vi "Dialog_SelectTarget.vi"(5 "error in (no error)":errorcluster) -> (15 "target address out":string, 16 "cancel?":bool, 17 "TCP port out":u16, 19 "error out":errorcluster)   [LabVIEW 2017, in "G#RemoteProxy.lvclass"]
doc: "Dialog that let you select the target to debug."
uses:
  G#RemoteProxy.lvclass
panel:
  in  "TCP Port":u16=62001
  in  "Available Targets":i32(ring) items=["My Computer (0.0.0.0)"]
  in  "TargetType":enum32{"Targets in project", "Specify"}(radio)
  in  "Cancel":bool
  in  "Specify target address":string
  in  "Connect":bool
  # "Select Target"
  # "Make sure that the\nG#DebugServer is running\non the remote target."
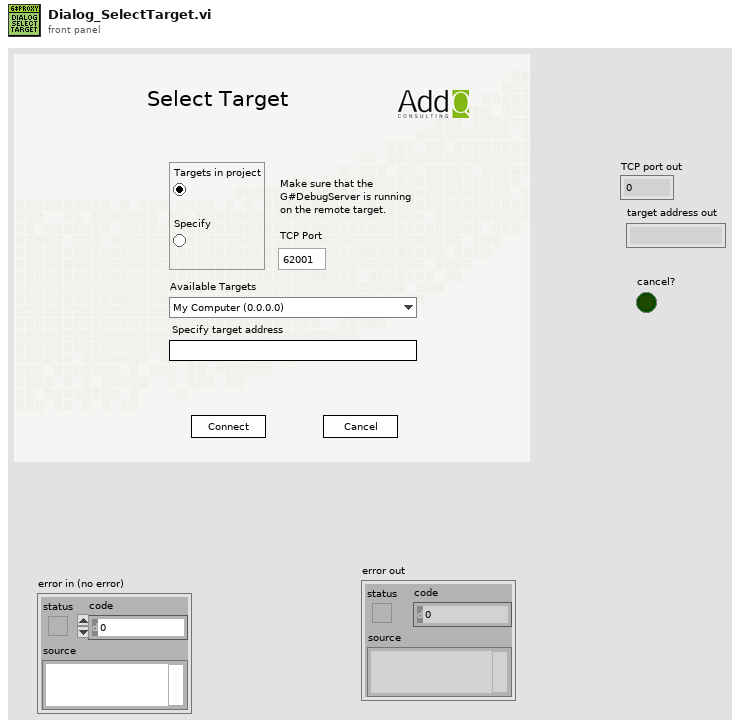
[diagram p1: front panel]
types:
  T1 = enum8{"Enabled", "Disabled", "Disabled and Grayed Out"}
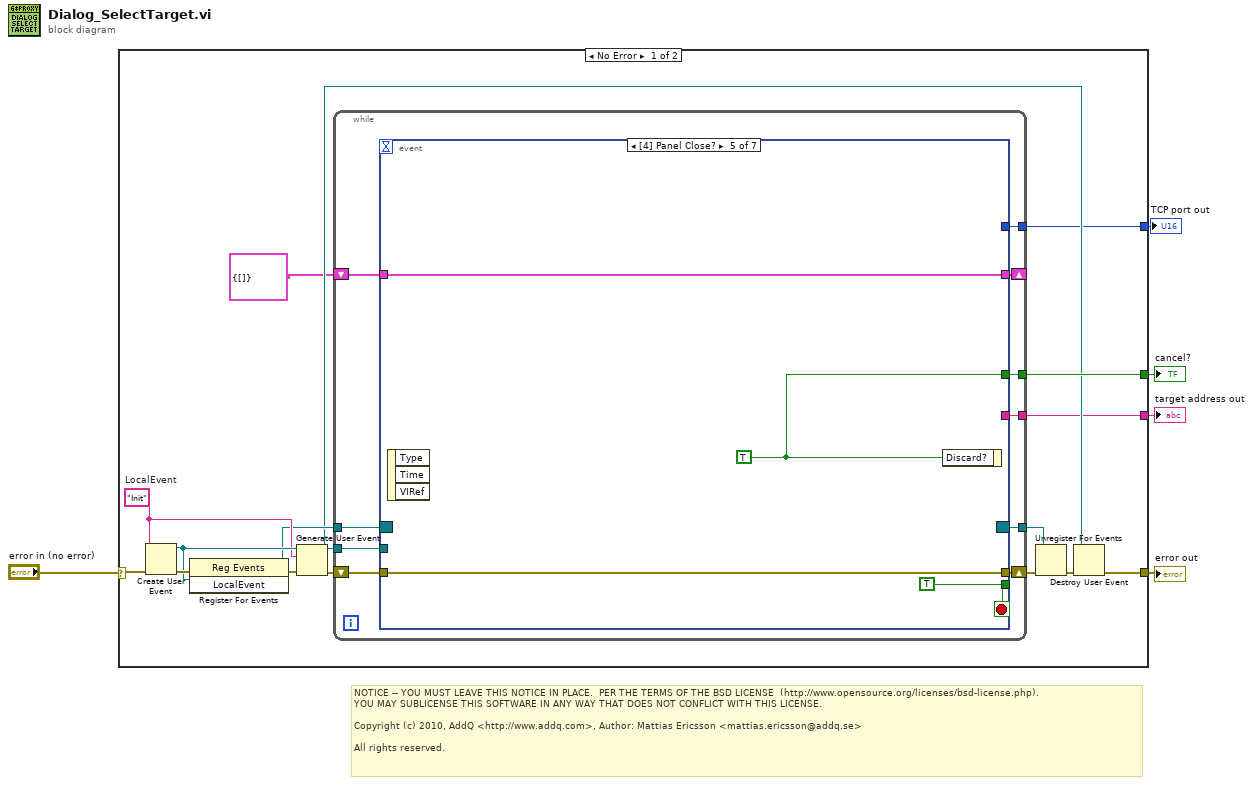
[diagram p0: block diagram]
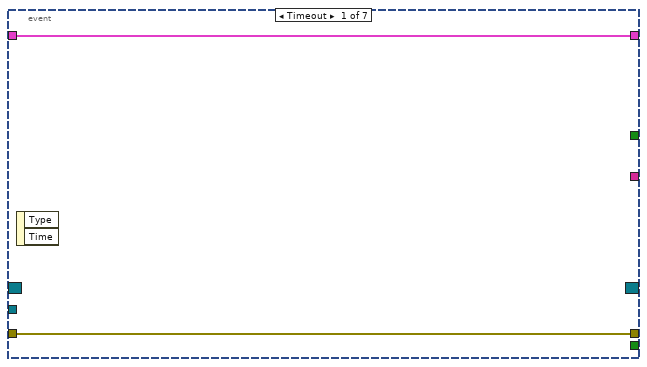
[diagram p2: hidden frame]
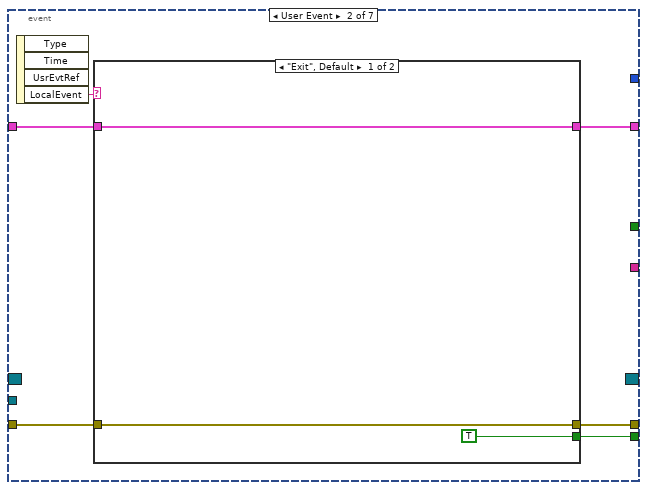
[diagram p3: hidden frame]
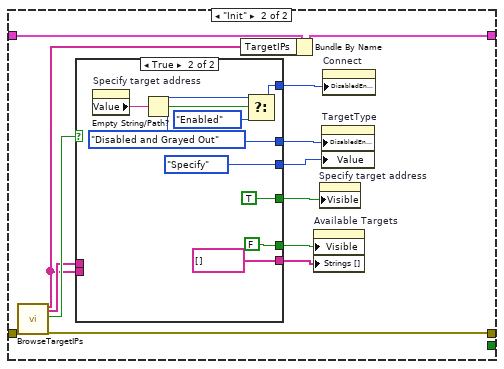
[diagram p4: hidden frame]
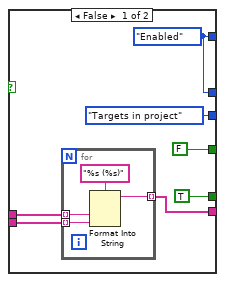
[diagram p5: hidden frame]
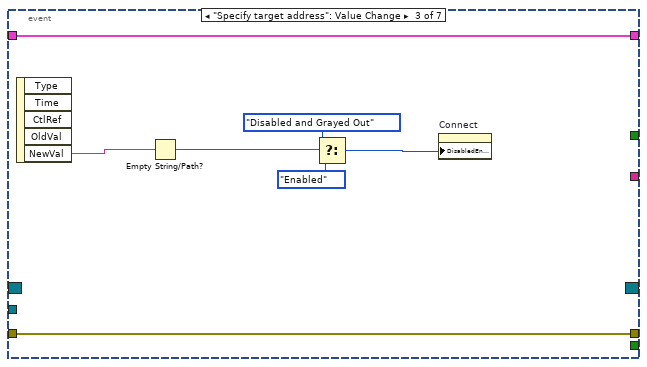
[diagram p6: hidden frame]
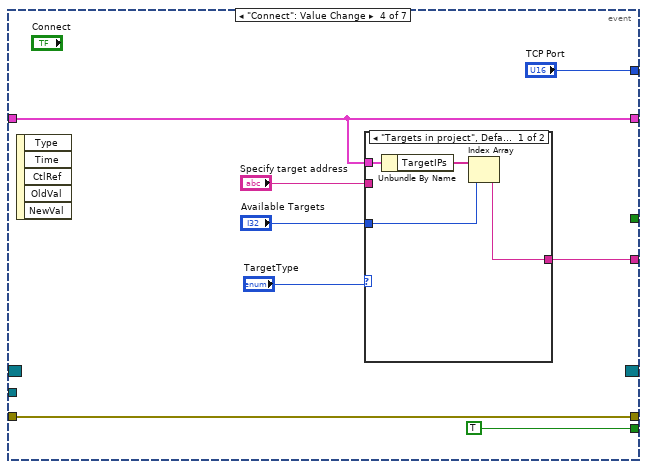
[diagram p7: hidden frame]
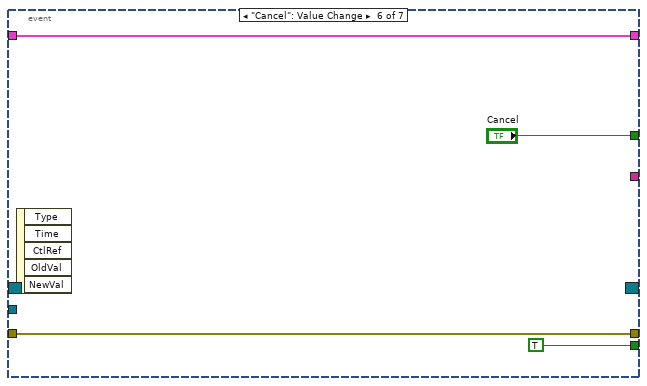
[diagram p9: hidden frame]
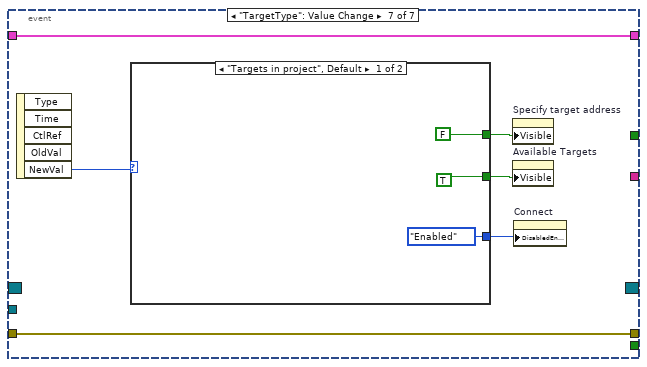
[diagram p10: hidden frame]
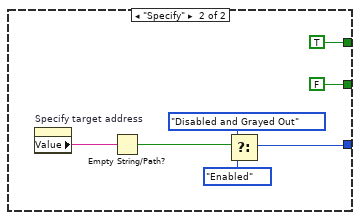
[diagram p11: hidden frame]
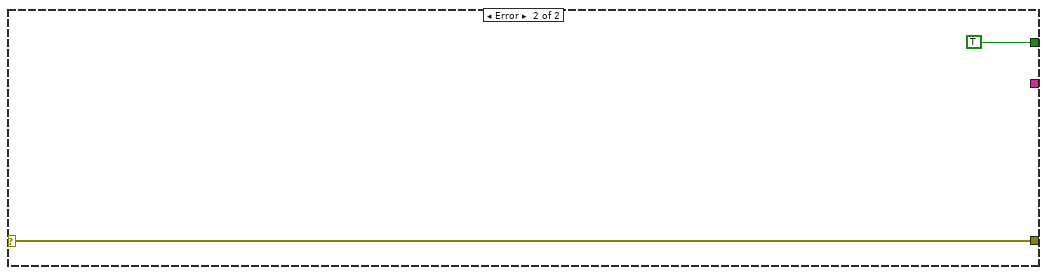
[diagram p12: hidden frame]
diagram:
  # "NOTICE -- YOU MUST LEAVE THIS NOTICE IN PLACE.  PER THE TERMS OF THE BSD LICENSE  (http://www.opensource.org/licenses/bsd-license.php).\nYOU MAY SUBLICENSE THIS SOFTWARE IN ANY WAY THAT DOES NOT CONFLICT WITH THIS LICENSE.\n\nCopyright (c) 2010, AddQ <http://www.addq.com>, Author: Mattias Ericsson <mattias.ericsson@addq.se>\n\nAll rights reserved."
  n1 = case shown="No Error" "error in (no error)" {
    selector: "error in (no error)" -> [w7 w122]
    tunnel: [w21 TRUE ("Cancel")] -> w5
    tunnel: [w9 _] -> w4
    tunnel: [w8 w122] -> w3
    tunnel: [w6 _] -> w1
    frame No Error {
      w16 = "Init"  # LocalEvent
      n2 = Create User Event(user event datatype=w16, error in=w7) -> (user event=w17:refnum<user-event>, error out=w20:errorcluster)
      n3 = register-events(error in=w20, w17) -> (reference out=w15:refnum<event-registration>, error out=w18:errorcluster)  [unwired: 1 in]
      n4 = Generate User Event(user event=w17, event data cluster=w16, error in=w18) -> (user event out=w11:refnum<user-event>, error out=w19:errorcluster)  [unwired: 1 in]
      n5 = while {
        tunnel: [w29] -> w21
        shift-right: [w30] -> w14
        shift-left: w19 -> [w31]
        tunnel: w15 -> [w28]
        tunnel: [w27] -> w13
        tunnel: w11 -> [w26]
        shift-right: [w24] -> _
        shift-left: cluster{"TargetIPs":string[]} {"TargetIPs"=[]} -> [w25]
        tunnel: [w23] -> w9
        tunnel: [w22] -> w6
        stop <- w32 stop-if-true
        n6 = event shown="[4] Panel Close?" {
          selector: w28 -> [_ _ _ _ _ _ _]
          dyn-events: [_ _ _ _ _ _ _] -> w27
          timeout: _ -> [_ _ _ _ _ _ _]
          tunnel: [_ w37 _ TRUE TRUE TRUE _] -> w32
          tunnel: w31 -> [w34 w40 w83 w90 w99 w103 w110]
          tunnel: [w34 w38 w83 w90 w99 w103 w110] -> w30
          tunnel: [_ _ _ _ w98 "Cancel" _] -> w29
          tunnel: w26 -> [_ _ _ _ _ _ _]
          tunnel: w25 -> [w33 w36 w82 w86 w97 w101 w109]
          tunnel: [w33 w35 w82 w86 w97 w101 w109] -> w24
          tunnel: [_ _ _ w87 _ _ _] -> w23
          tunnel: [_ _ _ "TCP Port" _ _ _] -> w22
          event Timeout {
            n7 = event-data() -> ()  [unwired: 1 in, 2 out]
          }
          event User Event {
            n8 = event-data() -> ("LocalEvent"=w39:string)  [unwired: 1 in, 3 out]
            n9 = case shown="\"Exit\", Default" w39 {
              tunnel: w40 -> [w43 w56]
              tunnel: [w43 w47] -> w38
              tunnel: [TRUE _] -> w37
              tunnel: w36 -> [w41 w50]
              tunnel: [w41 w45] -> w35
              frame "Exit", Default {
              }
              frame "Init" {
                n10 = call "BrowseTargetIPs.vi"("error in (no error)"=w56) -> ("target IPs"=w48:string[], "target names"=w49:string[], "no targets?"=w55:bool, "error out"=w47:errorcluster)  [unwired: 15 in]
                n11 = case shown="True" w55 {
                  tunnel: [w57 w71] -> w54
                  tunnel: [enum32{"Targets in project", "Specify"}."Targets in project" ("TargetType") enum32{"Targets in project", "Specify"}."Specify" ("TargetType")] -> w53
                  tunnel: [FALSE TRUE] -> w52
                  tunnel: [TRUE FALSE] -> w51
                  tunnel: w49 -> [w60 _]
                  tunnel: w48 -> [w59 _]
                  tunnel: [w58 string[] []] -> w46
                  tunnel: [w57 w68] -> w44
                  frame False {
                    w57 = T1."Enabled" ("Disabled")
                    n12 = for {
                      tunnel: w60 -> [w66] mode=indexing
                      tunnel: w59 -> [w65] mode=indexing
                      tunnel: [w64] -> w58 mode=indexing
                      n13 = Format Into String(format string="%s (%s)", w66, w65) -> (resulting string=w64:string)  [unwired: 2 in, 1 out]
                    }
                  }
                  frame True {
                    w71 = T1."Disabled and Grayed Out" ("Disabled")
                    n14 = property on="Specify target address" class="Str"() -> ("Value"=w72:string)  [unwired: 2 in, 2 out]
                    n15 = Empty String/Path?(string/path=w72) -> (empty?=w70:bool)
                    n16 = Select(t=w71, s=w70, f=T1."Enabled" ("Disabled")) -> (s? t:f=w68:T1)
                  }
                }
                n17 = Bundle By Name(cluster=w50, "TargetIPs"=w48) -> (w45:cluster{"TargetIPs":string[]})
                n18 = property on="Available Targets" class="Ring (strict)"("Visible"=w51, "Strings []"=w46) -> ()  [unwired: 2 in, 2 out]
                n19 = property on="Specify target address" class="Str"("Visible"=w52) -> ()  [unwired: 2 in, 2 out]
                n20 = property on="TargetType" class="RadioBtnsControl (strict)"("DisabledEnum"=w54, "Value"=w53) -> ()  [unwired: 2 in, 2 out]
                n21 = property on="Connect" class="Bool"("DisabledEnum"=w44) -> ()  [unwired: 2 in, 2 out]
              }
            }
          }
          event "Specify target address": Value Change {
            n22 = event-data() -> ("NewVal"=w78:string)  [unwired: 1 in, 4 out]
            n23 = Empty String/Path?(string/path=w78) -> (empty?=w80:bool)
            n24 = Select(t=T1."Disabled and Grayed Out" ("Disabled"), s=w80, f=T1."Enabled" ("Disabled")) -> (s? t:f=w77:T1)
            n25 = property on="Connect" class="Bool"("DisabledEnum"=w77) -> ()  [unwired: 2 in, 2 out]
          }
          event "Connect": Value Change {
            n26 = event-data() -> ()  [unwired: 1 in, 5 out]
            n27 = case shown="\"Targets in project\", Default" "TargetType" {
              tunnel: "Specify target address" -> [_ w96]
              tunnel: [w92 w96] -> w87
              tunnel: w86 -> [w95 _]
              tunnel: "Available Targets" -> [w94 _]
              frame "Targets in project", Default {
                n28 = Unbundle By Name(w95) -> ("TargetIPs"=w93:string[])
                n29 = Index Array(array=w93, index=w94) -> (element=w92:string)
              }
              frame "Specify" {
              }
            }
          }
          event Panel Close? {
            w98 = TRUE ("Discard?")
            n30 = event-data() -> ()  [unwired: 1 in, 3 out]
            n31 = event-data("Discard?"=w98) -> ()  [unwired: 1 in, 1 out]
          }
          event "Cancel": Value Change {
            n32 = event-data() -> ()  [unwired: 1 in, 5 out]
          }
          event "TargetType": Value Change {
            n33 = event-data() -> ("NewVal"=w108:enum32{"Targets in project", "Specify"})  [unwired: 1 in, 4 out]
            n34 = case shown="\"Targets in project\", Default" w108 {
              tunnel: [TRUE FALSE] -> w107
              tunnel: [FALSE TRUE] -> w106
              tunnel: [T1."Enabled" ("Disabled") w115] -> w105
              frame "Targets in project", Default {
              }
              frame "Specify" {
                n35 = property on="Specify target address" class="Str"() -> ("Value"=w118:string)  [unwired: 2 in, 2 out]
                n36 = Empty String/Path?(string/path=w118) -> (empty?=w117:bool)
                n37 = Select(t=T1."Disabled and Grayed Out" ("Disabled"), s=w117, f=T1."Enabled" ("Disabled")) -> (s? t:f=w115:T1)
              }
            }
            n38 = property on="Specify target address" class="Str"("Visible"=w106) -> ()  [unwired: 2 in, 2 out]
            n39 = property on="Available Targets" class="Ring (strict)"("Visible"=w107) -> ()  [unwired: 2 in, 2 out]
            n40 = property on="Connect" class="Bool"("DisabledEnum"=w105) -> ()  [unwired: 2 in, 2 out]
          }
        }
      }
      n41 = Unregister For Events(event registration refnum=w13, error in=w14) -> (error out=w12:errorcluster)
      n42 = Destroy User Event(user event=w11, error in=w12) -> (error out=w8:errorcluster)
    }
    frame Error {
    }
  }
  "error out" <- w3
  "cancel?" <- w5
  "target address out" <- w4
  "TCP port out" <- w1
